vi "Enqueue AppEvent Element.vi"(8 "Error In":errorcluster, 9 "Timeout":i32, 10 "Event Occured":refnum<class "Event.lvclass">, 11 "EventLog in":refnum<class "EventLog.lvclass">) -> (0 "Error Out":errorcluster, 1 "Timed out?":bool, 3 "EventLog out":refnum<class "EventLog.lvclass">)   [LabVIEW 2019, in "EventLog.lvlib" / "EventLog.lvclass"]
uses:
  EventLog.lvclass
  Classes/Event/Event.lvclass
  EventLog.lvclass/EventLog.ctl
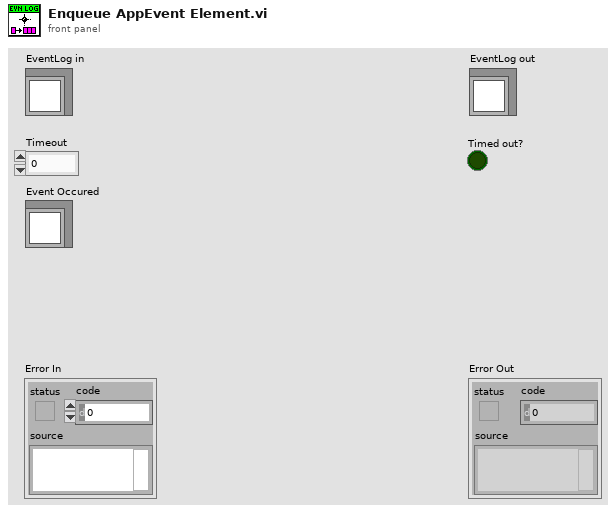
[diagram p1: front panel]
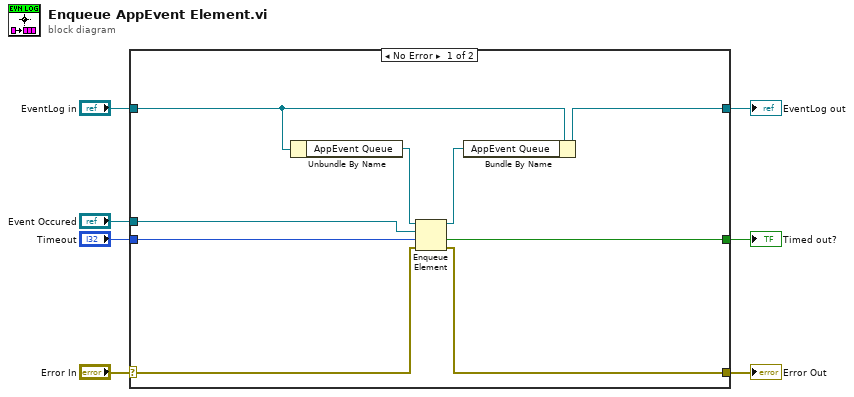
[diagram p0: block diagram]
diagram:
  n1 = case shown="No Error" "Error In" {
    selector: "Error In" -> [w14 w18]
    tunnel: [w9 w18] -> w6
    tunnel: [w13 w17] -> w4
    tunnel: "EventLog in" -> [w16 w17]
    tunnel: [w10 _] -> w3
    tunnel: "Timeout" -> [w11 _]
    tunnel: "Event Occured" -> [w8 _]
    frame No Error {
      n2 = Unbundle By Name(w16) -> ("AppEvent Queue"=w15:refnum<queue>)
      n3 = Enqueue Element(queue=w15, element=w8, timeout in ms (-1)=w11, error in (no error)=w14) -> (queue out=w12:refnum<queue>, timed out?=w10:bool, error out=w9:errorcluster)
      n4 = Bundle By Name(cluster=w16, "AppEvent Queue"=w12) -> (w13:refnum<class "EventLog.lvclass">)
    }
    frame Error {
    }
  }
  "Error Out" <- w6
  "EventLog out" <- w4
  "Timed out?" <- w3
